vi "HW_set_IO_ports_3-pos.vi"(1 "Sync capability":u8, 2 "Sync parameters cluster input":T2={"IO general config."=12, "IO 1 configuration"=1, "IO 2 configuration"=1, "IO 3 configuration"=0, "IO 4 configuration"=0, "Activate ext. RS-232"=0, "IO inversion config."=0}) -> (0 "Sync parameters cluster output":T1={"SYNC configuration"=12, "IO 1 configuration"=1, "IO 2 configuration"=1, "IO 3 configuration"=0, "IO 4 configuration"=0, "Activate ext. RS-232"=0, "IO inversion config."=0})   [LabVIEW 2018, in "Tracker.lvlib"]
uses:
  <vilib>/Utility/miscctls.llb/LVPointTypeDef.ctl
  Tracker.lvlib
panel:
  in  "IO 4 invert":bool caption="Swap High/Low"
  in  "IO 3 invert":bool caption="Swap High/Low"
  in  "IO 2 invert":bool caption="Swap High/Low"
  in  "IO 1 invert":bool caption="Swap High/Low"
  in  "IO 4":u16(ring)=1 items=["Out", "In"]
  in  "IO 3":u16(ring)=1 items=["Out", "In"]
  in  "IO 2":u16(ring) items=["Out", "In", "Sync (p)"]
  in  "IO 1":u16(ring) items=["Out", "In", "Sync (t)"]
  in  "Activate ext. RS-232":bool
  in  "Reset IO":bool
  in  "IO 4 start/stop":bool caption="Start or stop via incoming TTL pulse"
  in  "IO 3 start/stop":bool caption="Start or stop via incoming TTL pulse"
  in  "IO 2 start/stop":bool caption="Initiate outgoing TTL pulse"
  in  "IO 1 start/stop":bool caption="Initiate outgoing TTL pulse"
  in  "Exit":bool
  in  "Save Settings":bool
  in  "IO 4 zone":bool
  in  "IO 3 zone":bool
  in  "IO 2 sync":bool
  in  "IO 2 zone":bool=TRUE
  in  "IO 1 sync":bool
  in  "IO 1 zone":bool=TRUE
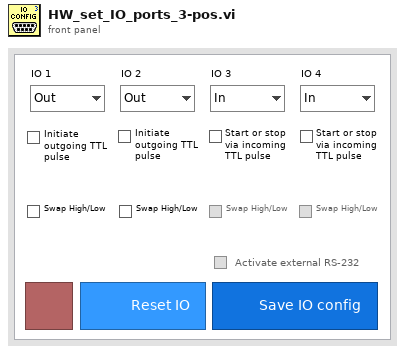
[diagram p1: front panel]
types:
  T1 = cluster{"SYNC configuration":u16, "IO 1 configuration":u16, "IO 2 configuration":u16, "IO 3 configuration":u16, "IO 4 configuration":u16, "Activate ext. RS-232":u16, "IO inversion config.":u16}
  T2 = cluster{"IO general config.":u16, "IO 1 configuration":u16, "IO 2 configuration":u16, "IO 3 configuration":u16, "IO 4 configuration":u16, "Activate ext. RS-232":u16, "IO inversion config.":u16}
  T3 = typedef "LVPointTypeDef.ctl" = cluster{"Horizontal":i16, "Vertical":i16}
  T4 = enum8{"Enabled", "Disabled", "Disabled and Grayed Out"}
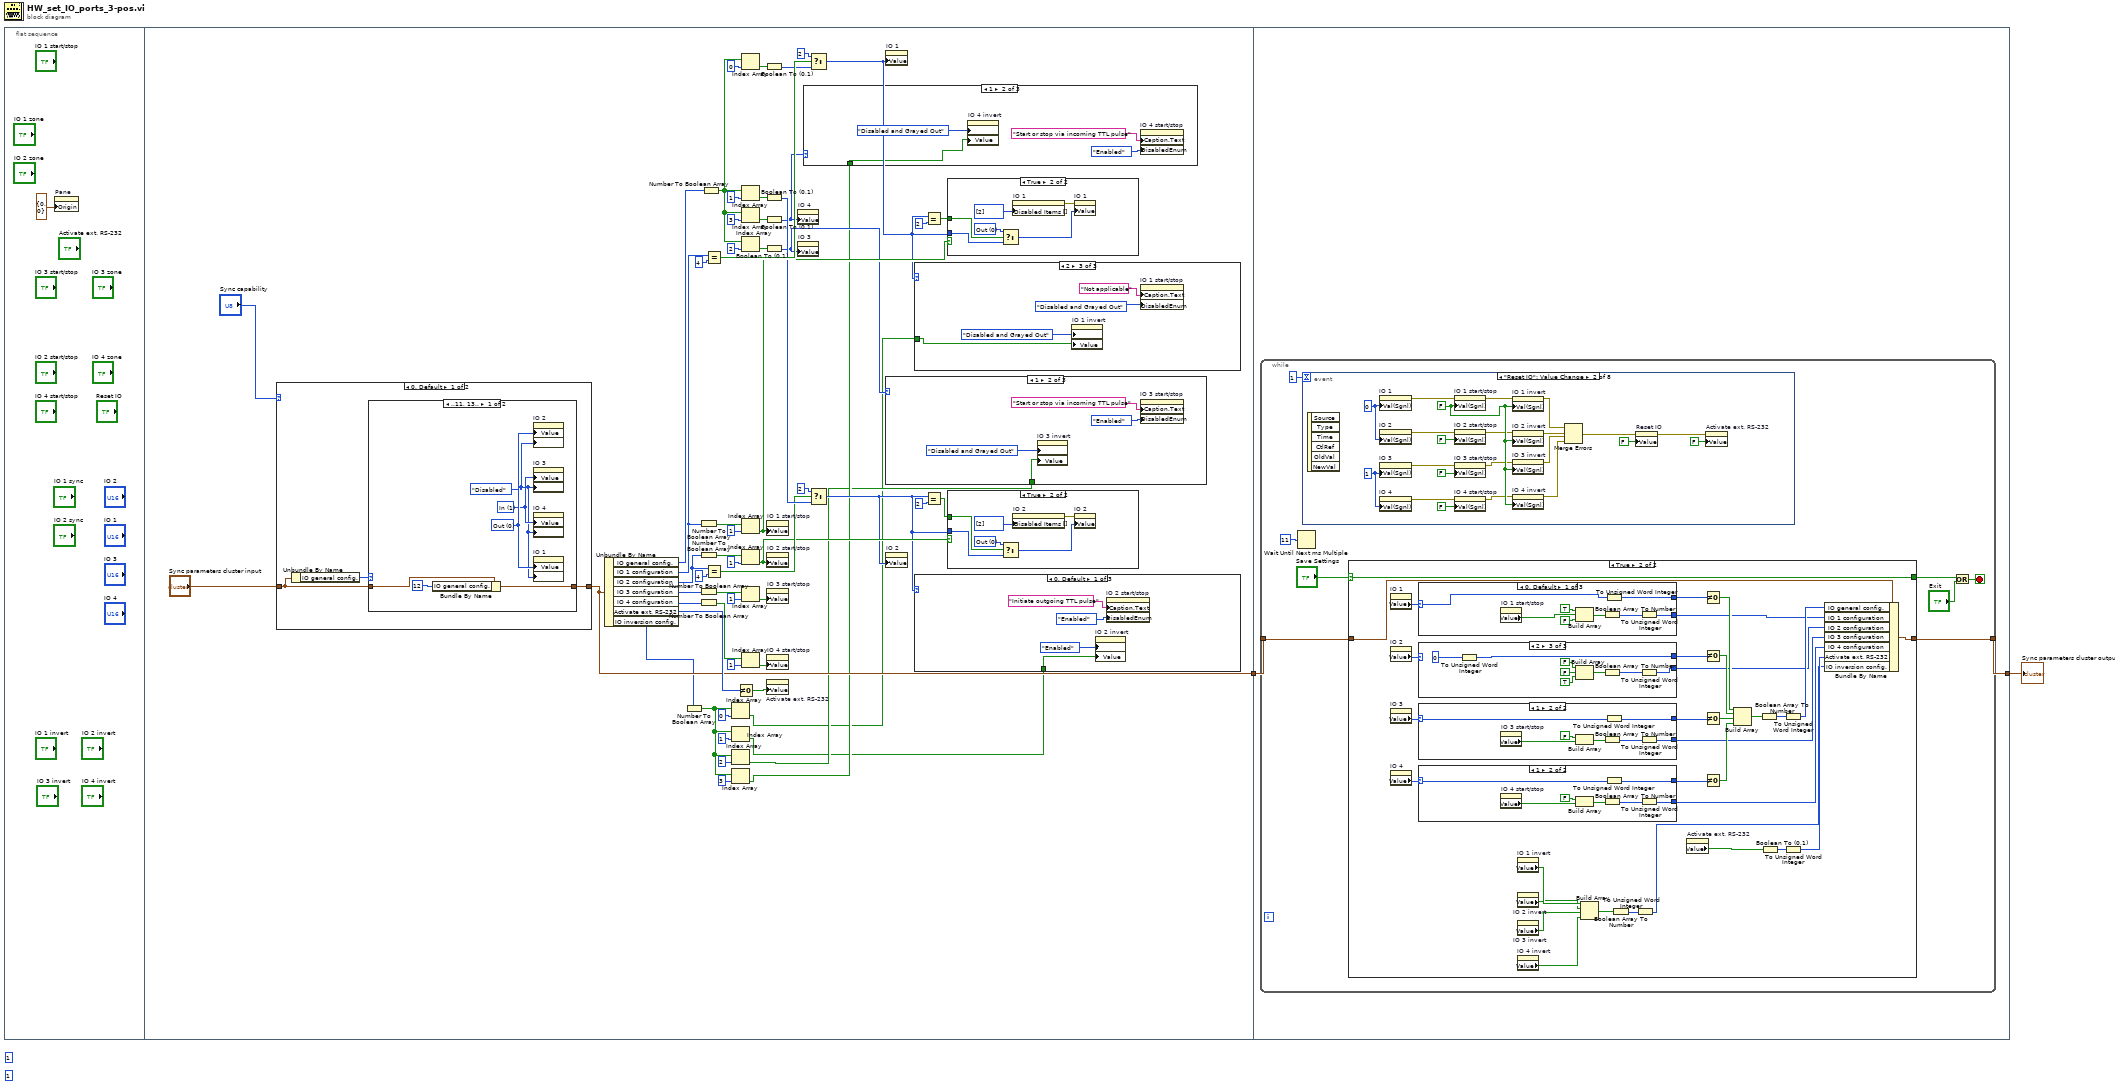
[diagram p0: block diagram]
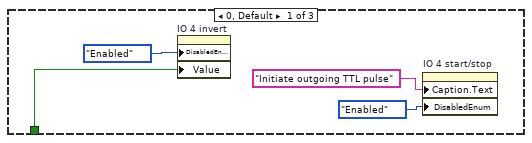
[diagram p2: hidden frame]
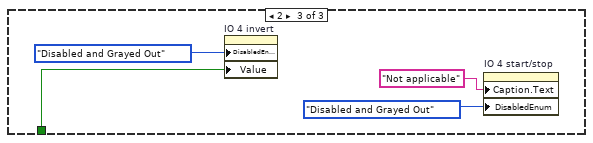
[diagram p3: hidden frame]
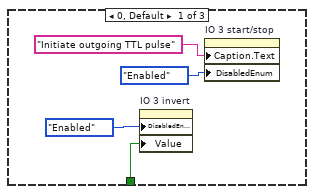
[diagram p4: hidden frame]
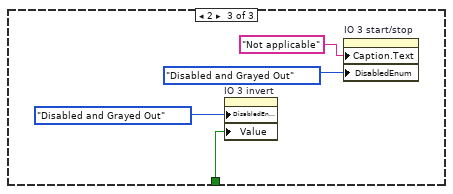
[diagram p5: hidden frame]
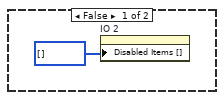
[diagram p6: hidden frame]
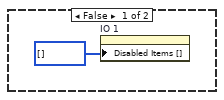
[diagram p7: hidden frame]
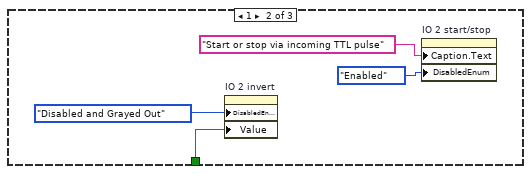
[diagram p8: hidden frame]
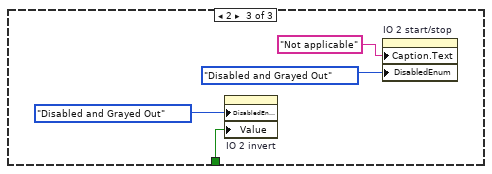
[diagram p9: hidden frame]
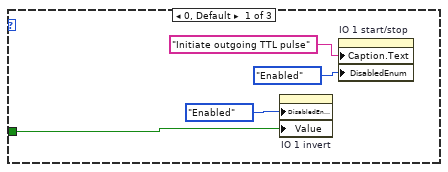
[diagram p10: hidden frame]
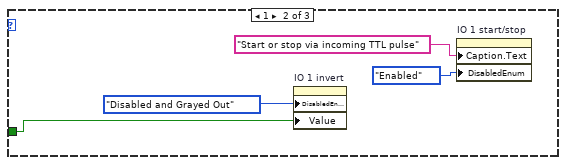
[diagram p11: hidden frame]
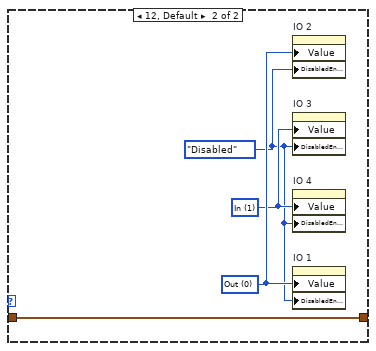
[diagram p12: hidden frame]
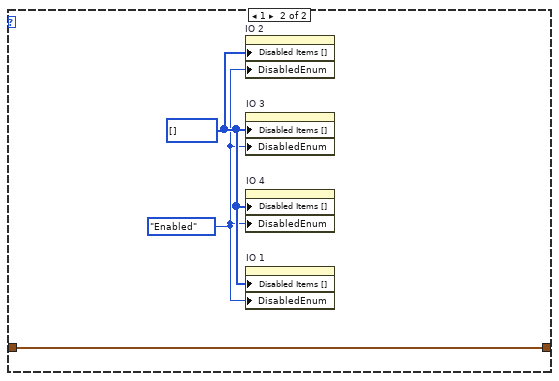
[diagram p13: hidden frame]
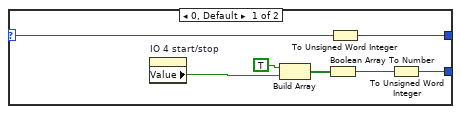
[diagram p15: hidden frame]
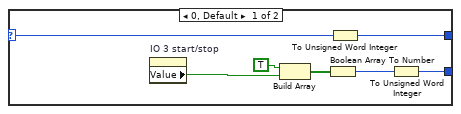
[diagram p16: hidden frame]
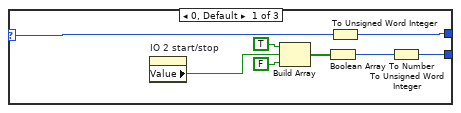
[diagram p17: hidden frame]
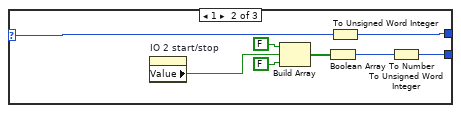
[diagram p18: hidden frame]
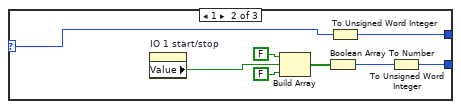
[diagram p19: hidden frame]
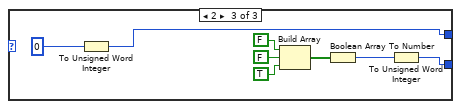
[diagram p20: hidden frame]
diagram:
  (unwired) 1 ("index")
  (unwired) 1 ("index")
  n1 = flat-sequence {
    tunnel: [w38] -> w2
    tunnel: [w140] -> w1
    tunnel: w2 -> [w139]
    frame #0 {
      n2 = property on="Pane" class="Pane"("Origin"=T3 {"Horizontal"=0, "Vertical"=0}) -> ()  [unwired: 2 in, 2 out]
    }
    frame #1 {
      n3 = case shown="0, Default" "Sync capability" {
        tunnel: "Sync parameters cluster input" -> [w124 w138]
        tunnel: [w123 w138] -> w38
        frame 0, Default {
          n4 = Unbundle By Name(w124) -> ("IO general config."=w125:u16)
          n5 = case shown="..11, 13.." w125 {
            tunnel: [w130 w135] -> w123
            tunnel: w124 -> [w131 w135]
            frame ..11, 13.. {
              w126 = T4."Disabled" ("Disabled")
              w127 = u16 1 items=["Out", "In"] ("IO 3")
              w128 = u16 0 items=["Out", "In", "Sync (t)"] ("IO 1")
              n6 = Bundle By Name(cluster=w131, "IO general config."=u16 12 ("SYNC configuration")) -> (w130:T2)
              n7 = property on="IO 2" class="Ring (strict)"("Value"=w128, "DisabledEnum"=w126) -> ()  [unwired: 2 in, 2 out]
              n8 = property on="IO 3" class="Ring (strict)"("Value"=w127, "DisabledEnum"=w126) -> ()  [unwired: 2 in, 2 out]
              n9 = property on="IO 4" class="Ring (strict)"("Value"=w127, "DisabledEnum"=w126) -> ()  [unwired: 2 in, 2 out]
              n10 = property on="IO 1" class="Ring (strict)"("Value"=w128, "DisabledEnum"=w126) -> ()  [unwired: 2 in, 2 out]
            }
            frame 12, Default {
              w132 = T4."Disabled" ("Disabled")
              w133 = u16 1 items=["Out", "In"] ("IO 3")
              w134 = u16 0 items=["Out", "In", "Sync (t)"] ("IO 1")
              n11 = property on="IO 2" class="Ring (strict)"("Value"=w134, "DisabledEnum"=w132) -> ()  [unwired: 2 in, 2 out]
              n12 = property on="IO 3" class="Ring (strict)"("Value"=w133, "DisabledEnum"=w132) -> ()  [unwired: 2 in, 2 out]
              n13 = property on="IO 4" class="Ring (strict)"("Value"=w133, "DisabledEnum"=w132) -> ()  [unwired: 2 in, 2 out]
              n14 = property on="IO 1" class="Ring (strict)"("Value"=w134, "DisabledEnum"=w132) -> ()  [unwired: 2 in, 2 out]
            }
          }
        }
        frame 1 {
          w136 = T4."Enabled" ("Disabled")
          w137 = i32[] [] ("Disabled Items []")
          n15 = property on="IO 2" class="Ring (strict)"("Disabled Items []"=w137, "DisabledEnum"=w136) -> ()  [unwired: 2 in, 2 out]
          n16 = property on="IO 3" class="Ring (strict)"("Disabled Items []"=w137, "DisabledEnum"=w136) -> ()  [unwired: 2 in, 2 out]
          n17 = property on="IO 4" class="Ring (strict)"("Disabled Items []"=w137, "DisabledEnum"=w136) -> ()  [unwired: 2 in, 2 out]
          n18 = property on="IO 1" class="Ring (strict)"("Disabled Items []"=w137, "DisabledEnum"=w136) -> ()  [unwired: 2 in, 2 out]
        }
      }
      n19 = Unbundle By Name(w38) -> ("IO general config."=w60:u16, "IO 1 configuration"=w33:u16, "IO 2 configuration"=w25:u16, "IO 3 configuration"=w44:u16, "IO 4 configuration"=w43:u16, "Activate ext. RS-232"=w42:u16, "IO inversion config."=w13:u16)
      n20 = Number To Boolean Array(number=w13) -> (Boolean array=w8:bool[])
      n21 = Number To Boolean Array(number=w33) -> (Boolean array=w50:bool[])
      n22 = Number To Boolean Array(number=w25) -> (Boolean array=w47:bool[])
      n23 = Number To Boolean Array(number=w44) -> (Boolean array=w46:bool[])
      n24 = Number To Boolean Array(number=w43) -> (Boolean array=w34:bool[])
      n25 = Number To Boolean Array(number=w60) -> (Boolean array=w59:bool[])
      n26 = Equal?(x=w33, y=u16 4) -> (x = y?=w31:bool)
      n27 = Equal?(x=w25, y=u16 4) -> (x = y?=w24:bool)
      n28 = Index Array(array=w8, index=0) -> (element=w4:bool)
      n29 = Index Array(array=w8, index=1) -> (element=w5:bool)
      n30 = Index Array(array=w8, index=2) -> (element=w6:bool)
      n31 = Index Array(array=w8, index=3) -> (element=w7:bool)
      n32 = Not Equal To 0?(x=w42) -> (x != 0?=w41:bool)
      n33 = Index Array(array=w59, index=0) -> (element=w54:bool)
      n34 = Index Array(array=w59, index=1) -> (element=w53:bool)
      n35 = Index Array(array=w59, index=3) -> (element=w51:bool)
      n36 = Index Array(array=w59, index=2) -> (element=w52:bool)
      n37 = Index Array(array=w50, index=1) -> (element=w22:bool)
      n38 = Index Array(array=w47, index=1) -> (element=w17:bool)
      n39 = Index Array(array=w46, index=1) -> (element=w45:bool)
      n40 = Index Array(array=w34, index=1) -> (element=w35:bool)
      n41 = Boolean To (0,1)(Boolean=w54) -> (0, 1=w30:i16)
      n42 = Boolean To (0,1)(Boolean=w53) -> (0, 1=w27:i16)
      n43 = Boolean To (0,1)(Boolean=w51) -> (0, 1=w14:i16)
      n44 = Boolean To (0,1)(Boolean=w52) -> (0, 1=w15:i16)
      n45 = property on="IO 1 start/stop" class="Bool (strict)"("Value"=w22) -> ()  [unwired: 2 in, 2 out]
      n46 = property on="IO 2 start/stop" class="Bool (strict)"("Value"=w17) -> ()  [unwired: 2 in, 2 out]
      n47 = property on="IO 3 start/stop" class="Bool (strict)"("Value"=w45) -> ()  [unwired: 2 in, 2 out]
      n48 = property on="IO 4 start/stop" class="Bool (strict)"("Value"=w35) -> ()  [unwired: 2 in, 2 out]
      n49 = property on="Activate ext. RS-232" class="Bool (strict)"("Value"=w41) -> ()  [unwired: 2 in, 2 out]
      n50 = property on="IO 4" class="Ring (strict)"("Value"=w14) -> ()  [unwired: 2 in, 2 out]
      n51 = property on="IO 3" class="Ring (strict)"("Value"=w15) -> ()  [unwired: 2 in, 2 out]
      n52 = case shown="1" w14 {
        tunnel: w7 -> [w61 w65 w69]
        frame 0, Default {
          n53 = property on="IO 4 invert" class="Bool (strict)"("DisabledEnum"=T4."Enabled" ("Disabled"), "Value"=w61) -> ()  [unwired: 2 in, 2 out]
          n54 = property on="IO 4 start/stop" class="Bool (strict)"("Caption.Text"="Initiate outgoing TTL pulse", "DisabledEnum"=T4."Enabled" ("Disabled")) -> ()  [unwired: 2 in, 2 out]
        }
        frame 1 {
          n55 = property on="IO 4 invert" class="Bool (strict)"("DisabledEnum"=T4."Disabled and Grayed Out" ("Disabled"), "Value"=w65) -> ()  [unwired: 2 in, 2 out]
          n56 = property on="IO 4 start/stop" class="Bool (strict)"("Caption.Text"="Start or stop via incoming TTL pulse", "DisabledEnum"=T4."Enabled" ("Disabled")) -> ()  [unwired: 2 in, 2 out]
        }
        frame 2 {
          n57 = property on="IO 4 invert" class="Bool (strict)"("DisabledEnum"=T4."Disabled and Grayed Out" ("Disabled"), "Value"=w69) -> ()  [unwired: 2 in, 2 out]
          n58 = property on="IO 4 start/stop" class="Bool (strict)"("Caption.Text"="Not applicable", "DisabledEnum"=T4."Disabled and Grayed Out" ("Disabled")) -> ()  [unwired: 2 in, 2 out]
        }
      }
      n59 = Select(t=i16 2, s=w31, f=w30) -> (s? t:f=w20:i16)
      n60 = Select(t=i16 2, s=w24, f=w27) -> (s? t:f=w16:i16)
      n61 = case shown="1" w15 {
        tunnel: w6 -> [w73 w77 w81]
        frame 0, Default {
          n62 = property on="IO 3 invert" class="Bool (strict)"("DisabledEnum"=T4."Enabled" ("Disabled"), "Value"=w73) -> ()  [unwired: 2 in, 2 out]
          n63 = property on="IO 3 start/stop" class="Bool (strict)"("Caption.Text"="Initiate outgoing TTL pulse", "DisabledEnum"=T4."Enabled" ("Disabled")) -> ()  [unwired: 2 in, 2 out]
        }
        frame 1 {
          n64 = property on="IO 3 invert" class="Bool (strict)"("DisabledEnum"=T4."Disabled and Grayed Out" ("Disabled"), "Value"=w77) -> ()  [unwired: 2 in, 2 out]
          n65 = property on="IO 3 start/stop" class="Bool (strict)"("Caption.Text"="Start or stop via incoming TTL pulse", "DisabledEnum"=T4."Enabled" ("Disabled")) -> ()  [unwired: 2 in, 2 out]
        }
        frame 2 {
          n66 = property on="IO 3 invert" class="Bool (strict)"("DisabledEnum"=T4."Disabled and Grayed Out" ("Disabled"), "Value"=w81) -> ()  [unwired: 2 in, 2 out]
          n67 = property on="IO 3 start/stop" class="Bool (strict)"("Caption.Text"="Not applicable", "DisabledEnum"=T4."Disabled and Grayed Out" ("Disabled")) -> ()  [unwired: 2 in, 2 out]
        }
      }
      n68 = property on="IO 1" class="Ring (strict)"("Value"=w20) -> ()  [unwired: 2 in, 2 out]
      n69 = property on="IO 2" class="Ring (strict)"("Value"=w16) -> ()  [unwired: 2 in, 2 out]
      n70 = case shown="2" w20 {
        tunnel: w4 -> [w111 w115 w119]
        frame 0, Default {
          n71 = property on="IO 1 invert" class="Bool (strict)"("DisabledEnum"=T4."Enabled" ("Disabled"), "Value"=w111) -> ()  [unwired: 2 in, 2 out]
          n72 = property on="IO 1 start/stop" class="Bool (strict)"("Caption.Text"="Initiate outgoing TTL pulse", "DisabledEnum"=T4."Enabled" ("Disabled")) -> ()  [unwired: 2 in, 2 out]
        }
        frame 1 {
          n73 = property on="IO 1 invert" class="Bool (strict)"("DisabledEnum"=T4."Disabled and Grayed Out" ("Disabled"), "Value"=w115) -> ()  [unwired: 2 in, 2 out]
          n74 = property on="IO 1 start/stop" class="Bool (strict)"("Caption.Text"="Start or stop via incoming TTL pulse", "DisabledEnum"=T4."Enabled" ("Disabled")) -> ()  [unwired: 2 in, 2 out]
        }
        frame 2 {
          n75 = property on="IO 1 invert" class="Bool (strict)"("DisabledEnum"=T4."Disabled and Grayed Out" ("Disabled"), "Value"=w119) -> ()  [unwired: 2 in, 2 out]
          n76 = property on="IO 1 start/stop" class="Bool (strict)"("Caption.Text"="Not applicable", "DisabledEnum"=T4."Disabled and Grayed Out" ("Disabled")) -> ()  [unwired: 2 in, 2 out]
        }
      }
      n77 = case shown="0, Default" w16 {
        tunnel: w5 -> [w99 w103 w107]
        frame 0, Default {
          n78 = property on="IO 2 invert" class="Bool (strict)"("DisabledEnum"=T4."Enabled" ("Disabled"), "Value"=w99) -> ()  [unwired: 2 in, 2 out]
          n79 = property on="IO 2 start/stop" class="Bool (strict)"("Caption.Text"="Initiate outgoing TTL pulse", "DisabledEnum"=T4."Enabled" ("Disabled")) -> ()  [unwired: 2 in, 2 out]
        }
        frame 1 {
          n80 = property on="IO 2 invert" class="Bool (strict)"("DisabledEnum"=T4."Disabled and Grayed Out" ("Disabled"), "Value"=w103) -> ()  [unwired: 2 in, 2 out]
          n81 = property on="IO 2 start/stop" class="Bool (strict)"("Caption.Text"="Start or stop via incoming TTL pulse", "DisabledEnum"=T4."Enabled" ("Disabled")) -> ()  [unwired: 2 in, 2 out]
        }
        frame 2 {
          n82 = property on="IO 2 invert" class="Bool (strict)"("DisabledEnum"=T4."Disabled and Grayed Out" ("Disabled"), "Value"=w107) -> ()  [unwired: 2 in, 2 out]
          n83 = property on="IO 2 start/stop" class="Bool (strict)"("Caption.Text"="Not applicable", "DisabledEnum"=T4."Disabled and Grayed Out" ("Disabled")) -> ()  [unwired: 2 in, 2 out]
        }
      }
      n84 = Equal?(x=w20, y=u16 2) -> (x = y?=w23:bool)
      n85 = Equal?(x=w16, y=u16 2) -> (x = y?=w19:bool)
      n86 = case shown="True" w22 {
        tunnel: w23 -> [_ w96]
        tunnel: w20 -> [_ w93]
        frame False {
          n87 = property on="IO 1" class="Ring (strict)"("Disabled Items []"=i32[] []) -> ()  [unwired: 2 in, 2 out]
        }
        frame True {
          w95 = u16 0 items=["Out", "In", "Sync (t)"] ("IO 1")
          n88 = Select(t=w95, s=w96, f=w93) -> (s? t:f=w94:u16)
          n89 = property on="IO 1" class="Ring (strict)"("Disabled Items []"=i32[] [2]) -> (error out=w97:errorcluster)  [unwired: 2 in, 1 out]
          n90 = property on="IO 1" class="Ring (strict)"(error in=w97, "Value"=w94) -> ()  [unwired: 1 in, 2 out]
        }
      }
      n91 = case shown="True" w17 {
        tunnel: w19 -> [_ w89]
        tunnel: w16 -> [_ w86]
        frame False {
          n92 = property on="IO 2" class="Ring (strict)"("Disabled Items []"=i32[] []) -> ()  [unwired: 2 in, 2 out]
        }
        frame True {
          w88 = u16 0 items=["Out", "In", "Sync (t)"] ("IO 1")
          n93 = Select(t=w88, s=w89, f=w86) -> (s? t:f=w87:u16)
          n94 = property on="IO 2" class="Ring (strict)"("Disabled Items []"=i32[] [2]) -> (error out=w90:errorcluster)  [unwired: 2 in, 1 out]
          n95 = property on="IO 2" class="Ring (strict)"(error in=w90, "Value"=w87) -> ()  [unwired: 1 in, 2 out]
        }
      }
    }
    frame #2 {
      n96 = while {
        tunnel: [w142] -> w140
        tunnel: w139 -> [w141]
        stop <- w145 stop-if-true
        n97 = Wait Until Next ms Multiple(millisecond multiple=u32 11) -> ()  [unwired: 1 out]
        n98 = event shown="[1] \"Reset IO\": Value Change" {
          selector: _ -> [_ _ _ _ _ _ _ _]
          dyn-events: _ -> [_ _ _ _ _ _ _ _]
          timeout: 1 -> [_ _ _ _ _ _ _ _]
          event Timeout {
            n99 = event-data() -> ()  [unwired: 1 in, 3 out]
          }
          event "Reset IO": Value Change {
            w270 = u16 1 ("Value (Signaling)")
            w271 = u16 0 ("Value (Signaling)")
            w265 = FALSE ("Value (Signaling)")
            n100 = event-data() -> ()  [unwired: 1 in, 6 out]
            n101 = property on="IO 1" class="Ring (strict)"("Val(Sgnl)"=w271) -> (error out=w269:errorcluster)  [unwired: 2 in, 1 out]
            n102 = property on="IO 2" class="Ring (strict)"("Val(Sgnl)"=w271) -> (error out=w268:errorcluster)  [unwired: 2 in, 1 out]
            n103 = property on="IO 3" class="Ring (strict)"("Val(Sgnl)"=w270) -> (error out=w278:errorcluster)  [unwired: 2 in, 1 out]
            n104 = property on="IO 4" class="Ring (strict)"("Val(Sgnl)"=w270) -> (error out=w276:errorcluster)  [unwired: 2 in, 1 out]
            n105 = property on="IO 1 start/stop" class="Bool (strict)"(error in=w269, "Val(Sgnl)"=w265) -> (error out=w267:errorcluster)  [unwired: 1 in, 1 out]
            n106 = property on="IO 2 start/stop" class="Bool (strict)"(error in=w268, "Val(Sgnl)"=FALSE ("Value (Signaling)")) -> (error out=w264:errorcluster)  [unwired: 1 in, 1 out]
            n107 = property on="IO 3 start/stop" class="Bool (strict)"(error in=w278, "Val(Sgnl)"=FALSE ("Value (Signaling)")) -> (error out=w263:errorcluster)  [unwired: 1 in, 1 out]
            n108 = property on="IO 4 start/stop" class="Bool (strict)"(error in=w276, "Val(Sgnl)"=FALSE ("Value (Signaling)")) -> (error out=w262:errorcluster)  [unwired: 1 in, 1 out]
            n109 = property on="IO 1 invert" class="Bool (strict)"(error in=w267, "Val(Sgnl)"=w265) -> (error out=w266:errorcluster)  [unwired: 1 in, 1 out]
            n110 = property on="IO 2 invert" class="Bool (strict)"(error in=w264, "Val(Sgnl)"=w265) -> (error out=w261:errorcluster)  [unwired: 1 in, 1 out]
            n111 = property on="IO 3 invert" class="Bool (strict)"(error in=w263, "Val(Sgnl)"=w265) -> (error out=w260:errorcluster)  [unwired: 1 in, 1 out]
            n112 = property on="IO 4 invert" class="Bool (strict)"(error in=w262, "Val(Sgnl)"=w265) -> (error out=w259:errorcluster)  [unwired: 1 in, 1 out]
            n113 = Merge Errors(w266, w261, w260, w259) -> (w275:errorcluster)
            n114 = property on="Reset IO" class="Bool (strict)"(error in=w275, "Value"=FALSE ("Reset IO")) -> (error out=w272:errorcluster)  [unwired: 1 in, 1 out]
            n115 = property on="Activate ext. RS-232" class="Bool (strict)"(error in=w272, "Value"=FALSE ("Activate ext. RS-232")) -> ()  [unwired: 1 in, 2 out]
          }
          event "IO 1": Value Change {
            n116 = event-data() -> ("NewVal"=w281:u16)  [unwired: 1 in, 5 out]
            n117 = case shown="1" w281 {
              frame 0, Default {
                w283 = T4."Enabled" ("Disabled")
                n118 = property on="IO 1 start/stop" class="Bool (strict)"("Caption.Text"="Initiate outgoing TTL pulse", "DisabledEnum"=w283) -> ()  [unwired: 2 in, 2 out]
                n119 = property on="IO 1 invert" class="Bool (strict)"("DisabledEnum"=w283) -> ()  [unwired: 2 in, 2 out]
              }
              frame 1 {
                n120 = property on="IO 1 invert" class="Bool (strict)"("DisabledEnum"=T4."Disabled and Grayed Out" ("Disabled"), "Value"=FALSE ("IO 1 invert")) -> ()  [unwired: 2 in, 2 out]
                n121 = property on="IO 1 start/stop" class="Bool (strict)"("Caption.Text"="Start or stop via incoming TTL pulse", "DisabledEnum"=T4."Enabled" ("Disabled")) -> ()  [unwired: 2 in, 2 out]
              }
              frame 2 {
                w290 = T4."Disabled and Grayed Out" ("Disabled")
                n122 = property on="IO 1 start/stop" class="Bool (strict)"("Caption.Text"="Not applicable", "DisabledEnum"=w290) -> ()  [unwired: 2 in, 2 out]
                n123 = property on="IO 1 invert" class="Bool (strict)"("DisabledEnum"=w290, "Value"=FALSE ("IO 1 invert")) -> ()  [unwired: 2 in, 2 out]
              }
            }
            n124 = property on="IO 1 start/stop" class="Bool (strict)"("Val(Sgnl)"=FALSE ("IO 1 start/stop")) -> ()  [unwired: 2 in, 2 out]
          }
          event "IO 2": Value Change {
            n125 = event-data() -> ("NewVal"=w292:u16)  [unwired: 1 in, 5 out]
            n126 = case shown="2" w292 {
              frame 0, Default {
                w294 = T4."Enabled" ("Disabled")
                n127 = property on="IO 2 start/stop" class="Bool (strict)"("Caption.Text"="Initiate outgoing TTL pulse", "DisabledEnum"=w294) -> ()  [unwired: 2 in, 2 out]
                n128 = property on="IO 2 invert" class="Bool (strict)"("DisabledEnum"=w294) -> ()  [unwired: 2 in, 2 out]
              }
              frame 1 {
                n129 = property on="IO 2 start/stop" class="Bool (strict)"("Caption.Text"="Start or stop via incoming TTL pulse", "DisabledEnum"=T4."Enabled" ("Disabled")) -> ()  [unwired: 2 in, 2 out]
                n130 = property on="IO 2 invert" class="Bool (strict)"("DisabledEnum"=T4."Disabled and Grayed Out" ("Disabled"), "Value"=FALSE ("IO 1 invert")) -> ()  [unwired: 2 in, 2 out]
              }
              frame 2 {
                n131 = property on="IO 2 start/stop" class="Bool (strict)"("Caption.Text"="Not applicable", "DisabledEnum"=T4."Disabled and Grayed Out" ("Disabled")) -> ()  [unwired: 2 in, 2 out]
                n132 = property on="IO 2 invert" class="Bool (strict)"("DisabledEnum"=T4."Disabled and Grayed Out" ("Disabled"), "Value"=FALSE ("IO 1 invert")) -> ()  [unwired: 2 in, 2 out]
              }
            }
            n133 = property on="IO 2 start/stop" class="Bool (strict)"("Val(Sgnl)"=FALSE ("IO 1 start/stop")) -> ()  [unwired: 2 in, 2 out]
          }
          event "IO 3": Value Change {
            n134 = event-data() -> ("NewVal"=w304:u16)  [unwired: 1 in, 5 out]
            n135 = case shown="1" w304 {
              frame 0, Default {
                w306 = T4."Enabled" ("Disabled")
                n136 = property on="IO 3 start/stop" class="Bool (strict)"("Caption.Text"="Initiate outgoing TTL pulse", "DisabledEnum"=w306) -> ()  [unwired: 2 in, 2 out]
                n137 = property on="IO 3 invert" class="Bool (strict)"("DisabledEnum"=w306) -> ()  [unwired: 2 in, 2 out]
              }
              frame 1 {
                n138 = property on="IO 3 start/stop" class="Bool (strict)"("Caption.Text"="Start or stop via incoming TTL pulse", "DisabledEnum"=T4."Enabled" ("Disabled")) -> ()  [unwired: 2 in, 2 out]
                n139 = property on="IO 3 invert" class="Bool (strict)"("DisabledEnum"=T4."Disabled and Grayed Out" ("Disabled"), "Value"=FALSE ("IO 1 invert")) -> ()  [unwired: 2 in, 2 out]
              }
              frame 2 {
                n140 = property on="IO 3 start/stop" class="Bool (strict)"("Caption.Text"="Not applicable", "DisabledEnum"=T4."Disabled and Grayed Out" ("Disabled")) -> ()  [unwired: 2 in, 2 out]
                n141 = property on="IO 3 invert" class="Bool (strict)"("DisabledEnum"=T4."Disabled and Grayed Out" ("Disabled"), "Value"=FALSE ("IO 1 invert")) -> ()  [unwired: 2 in, 2 out]
              }
            }
            n142 = property on="IO 3 start/stop" class="Bool (strict)"("Val(Sgnl)"=FALSE ("IO 1 start/stop")) -> ()  [unwired: 2 in, 2 out]
          }
          event "IO 4": Value Change {
            n143 = event-data() -> ("NewVal"=w316:u16)  [unwired: 1 in, 5 out]
            n144 = case shown="0, Default" w316 {
              frame 0, Default {
                w318 = T4."Enabled" ("Disabled")
                n145 = property on="IO 4 start/stop" class="Bool (strict)"("Caption.Text"="Initiate outgoing TTL pulse", "DisabledEnum"=w318) -> ()  [unwired: 2 in, 2 out]
                n146 = property on="IO 4 invert" class="Bool (strict)"("DisabledEnum"=w318) -> ()  [unwired: 2 in, 2 out]
              }
              frame 1 {
                n147 = property on="IO 4 start/stop" class="Bool (strict)"("Caption.Text"="Start or stop via incoming TTL pulse", "DisabledEnum"=T4."Enabled" ("Disabled")) -> ()  [unwired: 2 in, 2 out]
                n148 = property on="IO 4 invert" class="Bool (strict)"("DisabledEnum"=T4."Disabled and Grayed Out" ("Disabled"), "Value"=FALSE ("IO 1 invert")) -> ()  [unwired: 2 in, 2 out]
              }
              frame 2 {
                n149 = property on="IO 4 start/stop" class="Bool (strict)"("Caption.Text"="Not applicable", "DisabledEnum"=T4."Disabled and Grayed Out" ("Disabled")) -> ()  [unwired: 2 in, 2 out]
                n150 = property on="IO 4 invert" class="Bool (strict)"("DisabledEnum"=T4."Disabled and Grayed Out" ("Disabled"), "Value"=FALSE ("IO 1 invert")) -> ()  [unwired: 2 in, 2 out]
              }
            }
            n151 = property on="IO 4 start/stop" class="Bool (strict)"("Val(Sgnl)"=FALSE ("IO 1 start/stop")) -> ()  [unwired: 2 in, 2 out]
          }
          event "IO 1 start/stop": Value Change {
            n152 = event-data() -> ("NewVal"=w329:bool)  [unwired: 1 in, 5 out]
            n153 = property on="IO 1" class="Ring (strict)"() -> ("Value"=w328:u16)  [unwired: 2 in, 2 out]
            n154 = Equal?(x=w328, y=u16 2) -> (x = y?=w330:bool)
            n155 = case shown="True" w329 {
              tunnel: w330 -> [_ w336]
              tunnel: w328 -> [_ w333]
              frame False {
                n156 = property on="IO 1" class="Ring (strict)"("Disabled Items []"=i32[] []) -> ()  [unwired: 2 in, 2 out]
              }
              frame True {
                w335 = u16 0 items=["Out", "In", "Sync (t)"] ("IO 1")
                n157 = Select(t=w335, s=w336, f=w333) -> (s? t:f=w334:u16)
                n158 = property on="IO 1" class="Ring (strict)"("Disabled Items []"=i32[] [2]) -> (error out=w337:errorcluster)  [unwired: 2 in, 1 out]
                n159 = property on="IO 1" class="Ring (strict)"(error in=w337, "Value"=w334) -> ()  [unwired: 1 in, 2 out]
              }
            }
          }
          event "IO 2 start/stop": Value Change {
            n160 = event-data() -> ("NewVal"=w340:bool)  [unwired: 1 in, 5 out]
            n161 = property on="IO 2" class="Ring (strict)"() -> ("Value"=w339:u16)  [unwired: 2 in, 2 out]
            n162 = Equal?(x=w339, y=u16 2) -> (x = y?=w341:bool)
            n163 = case shown="True" w340 {
              tunnel: w341 -> [_ w347]
              tunnel: w339 -> [_ w344]
              frame False {
                n164 = property on="IO 2" class="Ring (strict)"("Disabled Items []"=i32[] []) -> ()  [unwired: 2 in, 2 out]
              }
              frame True {
                w346 = u16 0 items=["Out", "In", "Sync (t)"] ("IO 1")
                n165 = Select(t=w346, s=w347, f=w344) -> (s? t:f=w345:u16)
                n166 = property on="IO 2" class="Ring (strict)"("Disabled Items []"=i32[] [2]) -> (error out=w348:errorcluster)  [unwired: 2 in, 1 out]
                n167 = property on="IO 2" class="Ring (strict)"(error in=w348, "Value"=w345) -> ()  [unwired: 1 in, 2 out]
              }
            }
          }
        }
        n168 = case shown="True" "Save Settings" {
          selector: "Save Settings" -> [w150 w182]
          tunnel: [w150 w182] -> w143
          tunnel: [w149 w177] -> w142
          tunnel: w141 -> [w149 w178]
          frame False {
          }
          frame True {
            n169 = property on="IO 1" class="Ring (strict)"() -> ("Value"=w179:u16)  [unwired: 2 in, 2 out]
            n170 = property on="IO 2" class="Ring (strict)"() -> ("Value"=w176:u16)  [unwired: 2 in, 2 out]
            n171 = property on="IO 3" class="Ring (strict)"() -> ("Value"=w175:u16)  [unwired: 2 in, 2 out]
            n172 = property on="IO 4" class="Ring (strict)"() -> ("Value"=w174:u16)  [unwired: 2 in, 2 out]
            n173 = case shown="0, Default" w179 {
              selector: w179 -> [w238 w246 _]
              tunnel: [w235 w243 w252] -> w162
              tunnel: [w237 w245 w255] -> w167
              frame 0, Default {
                n174 = property on="IO 1 start/stop" class="Bool (strict)"() -> ("Value"=w242:bool)  [unwired: 2 in, 2 out]
                n175 = Build Array(TRUE, w242, FALSE) -> (w239:bool[])
                n176 = Boolean Array To Number(Boolean array=w239) -> (number=w236:u32)
                n177 = To Unsigned Word Integer(number=w238) -> (unsigned 16bit integer=w237:u16)
                n178 = To Unsigned Word Integer(number=w236) -> (unsigned 16bit integer=w235:u16)
              }
              frame 1 {
                n179 = property on="IO 1 start/stop" class="Bool (strict)"() -> ("Value"=w250:bool)  [unwired: 2 in, 2 out]
                n180 = Build Array(FALSE, w250, FALSE) -> (w247:bool[])
                n181 = Boolean Array To Number(Boolean array=w247) -> (number=w244:u32)
                n182 = To Unsigned Word Integer(number=w246) -> (unsigned 16bit integer=w245:u16)
                n183 = To Unsigned Word Integer(number=w244) -> (unsigned 16bit integer=w243:u16)
              }
              frame 2 {
                n184 = To Unsigned Word Integer(number=u16 0) -> (unsigned 16bit integer=w255:u16)
                n185 = Build Array(FALSE, FALSE, TRUE) -> (w256:bool[])
                n186 = Boolean Array To Number(Boolean array=w256) -> (number=w253:u32)
                n187 = To Unsigned Word Integer(number=w253) -> (unsigned 16bit integer=w252:u16)
              }
            }
            n188 = case shown="2" w176 {
              selector: w176 -> [w214 w222 _]
              tunnel: [w211 w219 w228] -> w161
              tunnel: [w213 w221 w231] -> w166
              frame 0, Default {
                n189 = property on="IO 2 start/stop" class="Bool (strict)"() -> ("Value"=w218:bool)  [unwired: 2 in, 2 out]
                n190 = Build Array(TRUE, w218, FALSE) -> (w215:bool[])
                n191 = Boolean Array To Number(Boolean array=w215) -> (number=w212:u32)
                n192 = To Unsigned Word Integer(number=w214) -> (unsigned 16bit integer=w213:u16)
                n193 = To Unsigned Word Integer(number=w212) -> (unsigned 16bit integer=w211:u16)
              }
              frame 1 {
                n194 = property on="IO 2 start/stop" class="Bool (strict)"() -> ("Value"=w226:bool)  [unwired: 2 in, 2 out]
                n195 = Build Array(FALSE, w226, FALSE) -> (w223:bool[])
                n196 = Boolean Array To Number(Boolean array=w223) -> (number=w220:u32)
                n197 = To Unsigned Word Integer(number=w222) -> (unsigned 16bit integer=w221:u16)
                n198 = To Unsigned Word Integer(number=w220) -> (unsigned 16bit integer=w219:u16)
              }
              frame 2 {
                n199 = To Unsigned Word Integer(number=u16 0) -> (unsigned 16bit integer=w231:u16)
                n200 = Build Array(FALSE, FALSE, TRUE) -> (w232:bool[])
                n201 = Boolean Array To Number(Boolean array=w232) -> (number=w229:u32)
                n202 = To Unsigned Word Integer(number=w229) -> (unsigned 16bit integer=w228:u16)
              }
            }
            n203 = case shown="1" w175 {
              selector: w175 -> [w200 w207]
              tunnel: [w197 w204] -> w160
              tunnel: [w199 w206] -> w165
              frame 0, Default {
                n204 = property on="IO 3 start/stop" class="Bool (strict)"() -> ("Value"=w203:bool)  [unwired: 2 in, 2 out]
                n205 = Build Array(TRUE, w203) -> (w201:bool[])
                n206 = Boolean Array To Number(Boolean array=w201) -> (number=w198:u32)
                n207 = To Unsigned Word Integer(number=w200) -> (unsigned 16bit integer=w199:u16)
                n208 = To Unsigned Word Integer(number=w198) -> (unsigned 16bit integer=w197:u16)
              }
              frame 1 {
                n209 = property on="IO 3 start/stop" class="Bool (strict)"() -> ("Value"=w210:bool)  [unwired: 2 in, 2 out]
                n210 = Build Array(FALSE, w210) -> (w208:bool[])
                n211 = Boolean Array To Number(Boolean array=w208) -> (number=w205:u32)
                n212 = To Unsigned Word Integer(number=w207) -> (unsigned 16bit integer=w206:u16)
                n213 = To Unsigned Word Integer(number=w205) -> (unsigned 16bit integer=w204:u16)
              }
            }
            n214 = case shown="1" w174 {
              selector: w174 -> [w186 w193]
              tunnel: [w183 w190] -> w159
              tunnel: [w185 w192] -> w164
              frame 0, Default {
                n215 = property on="IO 4 start/stop" class="Bool (strict)"() -> ("Value"=w189:bool)  [unwired: 2 in, 2 out]
                n216 = Build Array(TRUE, w189) -> (w187:bool[])
                n217 = Boolean Array To Number(Boolean array=w187) -> (number=w184:u32)
                n218 = To Unsigned Word Integer(number=w186) -> (unsigned 16bit integer=w185:u16)
                n219 = To Unsigned Word Integer(number=w184) -> (unsigned 16bit integer=w183:u16)
              }
              frame 1 {
                n220 = property on="IO 4 start/stop" class="Bool (strict)"() -> ("Value"=w196:bool)  [unwired: 2 in, 2 out]
                n221 = Build Array(FALSE, w196) -> (w194:bool[])
                n222 = Boolean Array To Number(Boolean array=w194) -> (number=w191:u32)
                n223 = To Unsigned Word Integer(number=w193) -> (unsigned 16bit integer=w192:u16)
                n224 = To Unsigned Word Integer(number=w191) -> (unsigned 16bit integer=w190:u16)
              }
            }
            n225 = property on="IO 1 invert" class="Bool (strict)"() -> ("Value"=w157:bool)  [unwired: 2 in, 2 out]
            n226 = property on="IO 2 invert" class="Bool (strict)"() -> ("Value"=w156:bool)  [unwired: 2 in, 2 out]
            n227 = property on="IO 3 invert" class="Bool (strict)"() -> ("Value"=w155:bool)  [unwired: 2 in, 2 out]
            n228 = property on="IO 4 invert" class="Bool (strict)"() -> ("Value"=w154:bool)  [unwired: 2 in, 2 out]
            n229 = Build Array(w157, w156, w155, w154) -> (w152:bool[])
            n230 = Boolean Array To Number(Boolean array=w152) -> (number=w153:u32)
            n231 = To Unsigned Word Integer(number=w153) -> (unsigned 16bit integer=w151:u16)
            n232 = property on="Activate ext. RS-232" class="Bool (strict)"() -> ("Value"=w181:bool)  [unwired: 2 in, 2 out]
            n233 = Not Equal To 0?(x=w167) -> (x != 0?=w173:bool)
            n234 = Not Equal To 0?(x=w166) -> (x != 0?=w172:bool)
            n235 = Not Equal To 0?(x=w165) -> (x != 0?=w171:bool)
            n236 = Not Equal To 0?(x=w164) -> (x != 0?=w170:bool)
            n237 = Build Array(w173, w172, w171, w170) -> (w169:bool[])
            n238 = Boolean Array To Number(Boolean array=w169) -> (number=w168:u32)
            n239 = Boolean To (0,1)(Boolean=w181) -> (0, 1=w180:i16)
            n240 = To Unsigned Word Integer(number=w168) -> (unsigned 16bit integer=w163:u16)
            n241 = To Unsigned Word Integer(number=w180) -> (unsigned 16bit integer=w158:u16)
            n242 = Bundle By Name(cluster=w178, "IO general config."=w163, "IO 1 configuration"=w162, "IO 2 configuration"=w161, "IO 3 configuration"=w160, "IO 4 configuration"=w159, "Activate ext. RS-232"=w158, "IO inversion config."=w151) -> (w177:T2)
          }
        }
        n243 = Or(x=w143, y="Exit") -> (x .or. y?=w145:bool)
      }
    }
  }
  "Sync parameters cluster output" <- w1
